vi "ReadAllofMultiiTiff_IFDonly.vi"(3 "error in":errorcluster, 5 "file path":path=path "D:/Messungen/tillx5/20240807_tillx5_beadsmehrfarb/I16/I16_B1_Raw.tif") -> (0 "error out":errorcluster)   [LabVIEW 2011]
uses:
  TiffModules/IFD.ctl
  TiffModules/ReadTiffPage_next.vi
  TiffModules/GetTagValue_U64.vi
panel:
  out "Waveform Graph":u64[](graph)=[4096, 125304832, 208838656, 250605568, 501207040, 459440128, 542973952, 626507776, 668274688, 710041600, 751808512, 793575424, 877109248, 835342336, 918876160, 960643072, 1169477632, 1253011456, 1294778368, 1378312192, 1336545280, 1420079104, 1461846016, 1503612928, 1670680576, 1712447488, 1754214400, 1795981312, 1837748224, 1879515136, 1921282048, 1963048960, 2004815872, 2046582784, 2088349696, 2130116608, 2213650432, 2255417344, 2380718080, 2506018816, 2673086464, 2714853376, 2798387200, 2756620288, 2923687936, 2840154112, 2881921024, 3132522496, 3675492352, 3717259264, 3759026176, 3800793088, 3884326912, 3842560000, 3926093824, 4134928384, 4677898240, 4719665152, 4761432064, 4886732800, 4970266624, 4928499712, 5053800448, 5095567360, 5346168832, 5471469568, 5513236480, 5722071040, 5555003392, 5638537216, 5847371776, 5889138688, 6014439424, 6097973248, 6181507072, 6515642368, 6265040896, 6432108544, 6390341632, 6640943104, 6682710016, 6766243840, 6849777664, 7183912960, 6891544576, 6975078400, 7058612224, 7142146048, 7392747520, 7476281344, 7518048256, 7601582080, 7643348992, 7768649728, 7893950464, 7935717376, 8102785024, 8061018112, 8186318848, 8436920320, 8353386496, 8311619584, 8395153408, 8603987968, 8687521792, 8896356352, 8771055616, 8938123264, 9021657088, 9105190912, 9230491648, 9272258560, 9355792384, 9439326208, 9522860032, 9606393856, 9689927680, 9648160768, 9773461504, 9940529152, 10024062976, 10107596800, 10232897536, 10191130624, 10399965184, 10316431360, 10483499008, 10608799744, 10692333568, 10775867392, 10859401216, 10942935040, 11026468864, 11151769600, 11193536512, 11277070336, 11360604160, 11444137984, 11527671808, 11569438720, 11694739456, 11778273280, 11861807104, 11945340928, 12028874752, 12112408576, 12195942400, 12279476224, 12363010048, 12446543872, 12571844608, 12613611520, 12697145344, 12822446080, 12864212992, 12947746816, 13031280640, 13114814464, 13198348288, 13281882112, 13407182848, 13448949760, 13532483584, 13616017408, 13699551232, 13783085056, 13866618880, 13950152704, 14033686528, 14158987264, 14200754176, 14284288000, 14367821824, 14451355648, 14534889472, 14618423296, 14701957120, 14785490944, 14869024768, 14952558592, 15036092416, 15119626240, 15203160064, 15286693888, 15370227712, 15453761536, 15537295360, 15620829184, 15704363008, 15787896832, 15871430656, 15954964480, 41771008, 83537920, 167071744, 292372480, 334139392, 417673216, 375906304, 584740864, 1002409984, 1044176896, 1085943808, 1127710720, 1211244544, 1545379840, 1587146752, 1628913664, 2171883520, 2297184256, 2338951168, 2422484992, 2464251904, 2547785728, 2589552640, 2631319552, 2965454848, 3007221760, 3048988672, 3090755584, 3174289408, 3257823232, 3216056320, 3299590144, 3341357056, 3383123968, 3424890880, 3508424704, 3466657792, 3550191616, 3591958528, 3633725440, 3967860736, 4009627648, 4093161472, 4051394560, 4218462208, 4176695296, 4301996032, 4260229120, 4343762944, 4385529856, 4427296768, 4469063680, 4510830592, 4552597504, 4594364416, 4636131328, 4803198976, 4844965888, 5012033536, 5137334272, 5179101184, 5220868096, 5262635008, 5304401920, 5387935744, 5680304128, 5429702656, 5972672512, 5596770304, 5805604864, 5763837952, 5930905600, 6056206336, 6139740160, 6223273984, 6306807808, 6348574720, 6473875456, 6557409280, 6599176192, 6724476928, 6808010752, 7016845312, 7100379136, 6933311488, 7267446784, 7225679872, 7309213696, 7350980608, 7434514432, 7559815168, 7726882816, 7685115904, 7810416640, 7852183552, 7977484288, 8019251200, 8228085760, 8144551936, 8269852672, 8520454144, 8478687232, 8562221056, 8645754880, 8729288704, 8854589440, 8812822528, 8979890176, 9063424000, 9146957824, 9188724736, 9314025472, 9397559296, 9481093120, 9564626944, 9898762240, 9982296064, 9815228416, 9731694592, 9856995328, 10065829888, 10149363712, 10441732096, 10274664448, 10358198272, 10525265920, 10567032832, 10650566656, 10734100480, 10817634304, 10901168128, 10984701952, 11068235776, 11110002688, 11235303424, 11318837248, 11402371072, 11485904896, 11611205632, 11652972544, 11736506368, 11820040192, 11903574016, 11987107840, 12070641664, 12154175488, 12237709312, 12321243136, 12404776960, 12488310784, 12530077696, 12655378432, 12738912256, 12780679168, 12905979904, 12989513728, 13073047552, 13156581376, 13240115200, 13323649024, 13365415936, 13490716672, 13574250496, 13657784320, 13741318144, 13824851968, 13908385792, 13991919616, 14075453440, 14117220352, 14242521088, 14326054912, 14409588736, 14493122560, 14576656384, 14660190208, 14743724032, 14827257856, 14910791680, 14994325504, 15077859328, 15161393152, 15244926976, 15328460800, 15411994624, 15495528448, 15579062272, 15662596096, 15746129920, 15829663744, 15913197568, 15996731392]
  out "Directory Entries":T1[][](array[typedef])
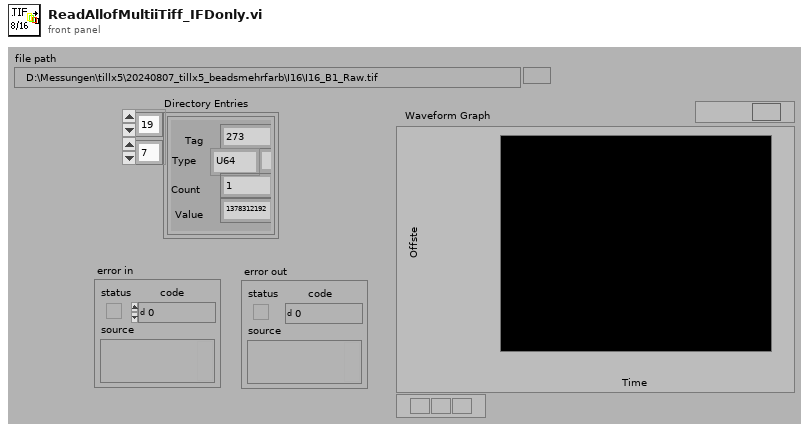
[diagram p1: front panel]
types:
  T1 = typedef "IFD.ctl" = cluster{"Tag":u16, "Type":enum16{"illegal", "Byte", "Ascii", "Short", "Long", "Rational", "SByte", "Undefined", "SShort", "SLong", "SRational 2xSLong", "Float 4byte", "Double 8Byte", "No13", "No14", "No15", "U64", "I64", "U64-IFD8"}, "Count":u64, "Value":u64}
  T2 = cluster{"Tiff refnum":refnum<file>, "BigTiff,Endian":u16}
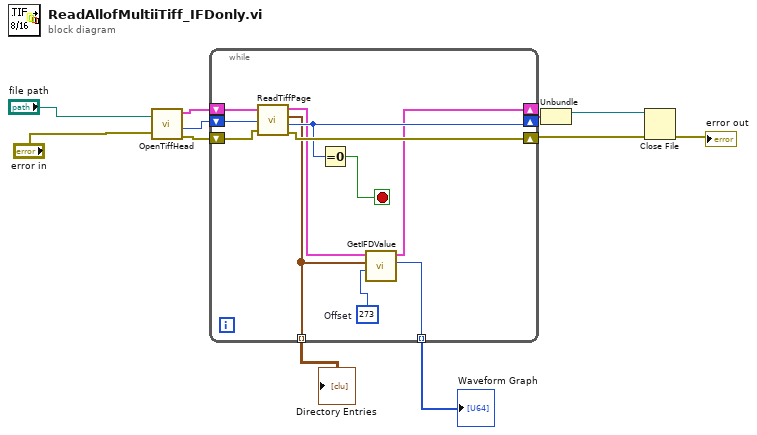
[diagram p0: block diagram]
diagram:
  n1 = call "OpenTiffHead.vi"("file path"="file path", "error in"="error in") -> ("TIFF file"=w8:T2, "first Diroffset"=w9:u64, "error out"=w7:errorcluster)  [unwired: 1 in]
  n2 = while {
    shift-right: [w18] -> _
    shift-left: w9 -> [w22]
    shift-right: [w13] -> w4
    shift-left: w8 -> [w21]
    shift-right: [w19] -> w3
    shift-left: w7 -> [w20]
    tunnel: [w16] -> w2 mode=indexing
    tunnel: [w12] -> w1 mode=indexing
    stop <- w17 stop-if-true
    w14 = u16 273  # Offset
    n3 = call-poly "ReadTiffPage.vi"("TIFF file"=w21, "IFDoffset"=w22, "error in"=w20) -> ("TIFF file out"=w15:T2, "Directory Entries"=w16:T1[], "Next offset"=w18:i64, "error out"=w19:errorcluster)  [unwired: 4 in]
    n4 = Equal To 0?(x=w18) -> (x = 0?=w17:bool)
    n5 = call-poly "GetIFDValue.vi"("Tag Code"=w14, "Directory Entries"=w16, "TIFF file"=w15) -> ("Single Value"=w12:u64, "TIFF file out"=w13:T2)  [unwired: 1 in, 4 out]
  }
  "Directory Entries" <- w2
  "Waveform Graph" <- w1
  n6 = Unbundle(w4) -> ("Tiff refnum"=w6:refnum<file>)  [unwired: 1 out]
  n7 = Close File(refnum=w6, error in=w3) -> (error out=→"error out":errorcluster)  [unwired: 1 out]
